vi "sort.by.volume.type.vi"(11 "Array in":T1[](array[typedef])) -> (1 "end date":timestamp, 2 "start date":timestamp, 3 "Array":cluster{T1[]}[](array[cluster]))   [LabVIEW 2024]
uses:
  volume.object--cluster.ctl
  definitions/volume.type--enum.ctl
  15bd804e-f082-4d16-99e2-ed414d39ba84.vi
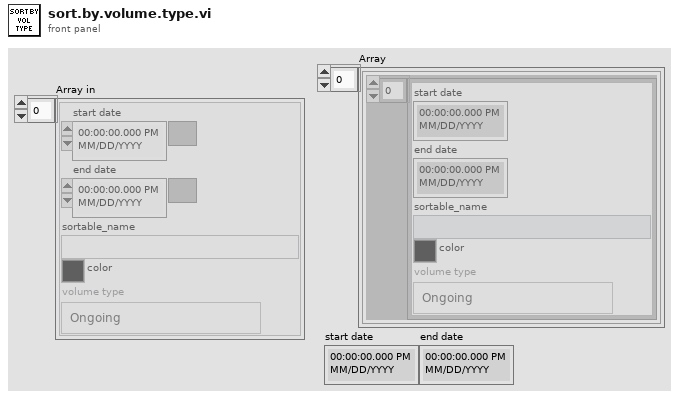
[diagram p1: front panel]
types:
  T1 = typedef "volume.object--cluster.ctl" = cluster{"start date":timestamp, "end date":timestamp, "sortable_name":string, "color":u32, "volume type":T2}
  T2 = typedef "volume.type--enum.ctl" = enum16{"Ongoing", "Limited Series", "Annual", "One Shot", "Reprint/Document"}
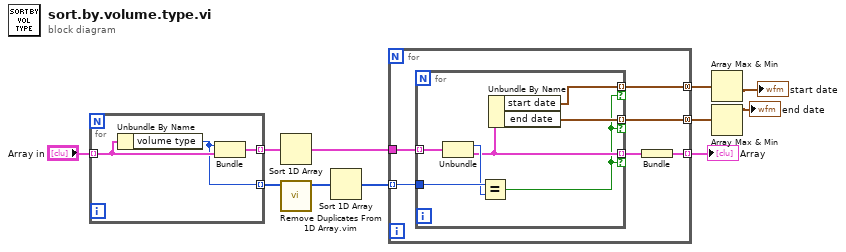
[diagram p0: block diagram]
diagram:
  n1 = for {
    tunnel: "Array in" -> [w14] mode=indexing
    tunnel: [w13] -> w10 mode=indexing
    tunnel: [w12] -> w8 mode=indexing
    n2 = Unbundle By Name(w14) -> ("volume type"=w12:T2)
    n3 = Bundle("volume type"=w12, "Cluster"=w14) -> (w13:cluster{"volume type":T2, "Cluster":T1})  [unwired: 1 in]
  }
  n4 = Sort 1D Array(array=w10) -> (sorted array=w11:cluster{"volume type":T2, "Cluster":T1}[])
  n5 = call "Remove Duplicates From 1D Array.vim"("array"=w8) -> ("array with duplicates removed"=w7:T2[])  [unwired: 10 in]
  n6 = Sort 1D Array(array=w7) -> (sorted array=w5:T2[])
  n7 = for {
    tunnel: [w17] -> w6 mode=indexing
    tunnel: w11 -> [w20]
    tunnel: w5 -> [w19] mode=indexing
    tunnel: [w16] -> w4 mode=concatenating
    tunnel: [w15] -> w2 mode=concatenating
    n8 = for {
      tunnel: w20 -> [w27] mode=indexing
      tunnel: [w24] -> w18 mode=indexing if=w21
      tunnel: w19 -> [w26]
      tunnel: [w23] -> w16 mode=indexing if=w21
      tunnel: [w22] -> w15 mode=indexing if=w21
      n9 = Unbundle(w27) -> ("volume type"=w25:T2, "Cluster"=w24:T1)
      n10 = Equal?(x=w26, y=w25) -> (x = y?=w21:bool)
      n11 = Unbundle By Name(w24) -> ("start date"=w23:timestamp, "end date"=w22:timestamp)
    }
    n12 = Bundle(w18) -> (w17:cluster{T1[]})  [unwired: 1 in]
  }
  "Array" <- w6
  n13 = Array Max & Min(array=w4) -> (min value=→"start date":timestamp)  [unwired: 3 out]
  n14 = Array Max & Min(array=w2) -> (max value=→"end date":timestamp)  [unwired: 3 out]
